vi "get image.vi"(8 "error in (no error)":errorcluster, 10 "previous buffer number":u32, 11 "image source data":T4) -> (0 "error out":errorcluster, 1 "aquisition time ms":u32, 2 "buffer number":u32, 3 "captured image":T1)   [LabVIEW 2013]
uses:
  <vilib>/userdefined/High Color/IMAQdx.ctl
  <vilib>/vision/Avi1.llb/AviRefnum.ctl
  <vilib>/vision/Image Controls.llb/IMAQ Image.ctl
  <vilib>/vision/driver/NI_Vision_Acquisition_Software.lvlib
  Image-Stack-Compressor/Stack Reader Wrapper/labview vis/StackReaderWrapper.lvlib
  <vilib>/vision/NI_Vision_Development_Module.lvlib
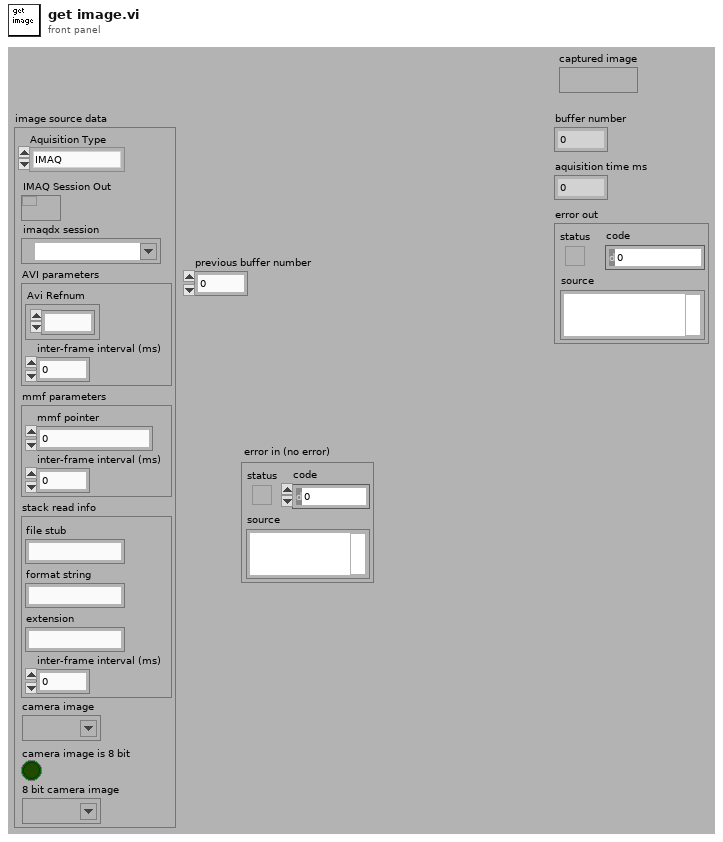
[diagram p1: front panel]
types:
  T1 = typedef "IMAQ Image.ctl" = refnum<image>
  T2 = typedef "IMAQdx.ctl" = refnum<k21>
  T3 = typedef "AviRefnum.ctl" = refnum<k1>
  T4 = cluster{"Aquisition Type":enum16{"IMAQ", "IMAQdx", "AVI", "MMF", "STACK"}, "IMAQ Session Out":refnum<k11>, "imaqdx session":T2, "AVI parameters":cluster{"Avi Refnum ":T3, "inter-frame interval (ms)":dbl}, "mmf parameters":cluster{"mmf pointer":u32, "inter-frame interval (ms)":dbl}, "stack read info":cluster{"file stub":string, "format string":string, "extension":string, "inter-frame interval (ms)":dbl}, "camera image":T1, "camera image is 8 bit":bool, "8 bit camera image":T1}
  T5 = cluster{"file stub":string, "format string":string, "extension":string, "inter-frame interval (ms)":dbl}
  T6 = typedef "Image Type" = u32
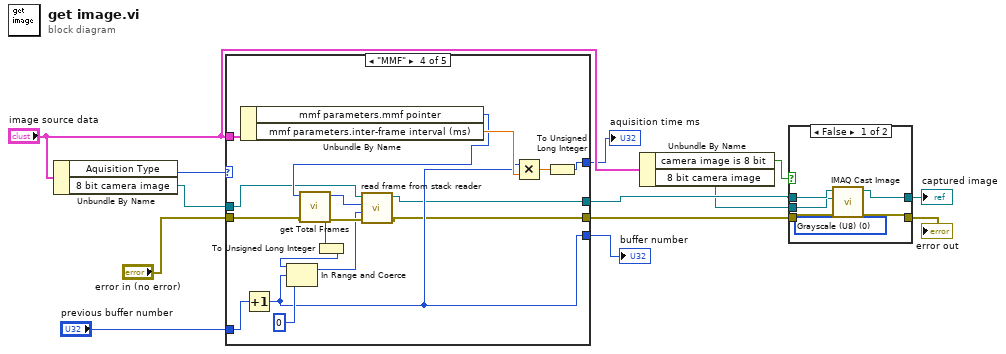
[diagram p0: block diagram]
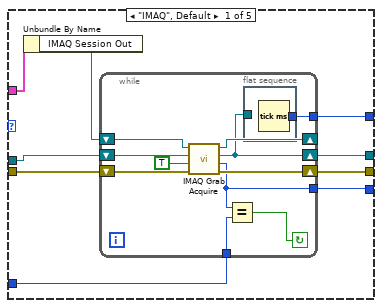
[diagram p3: hidden frame]
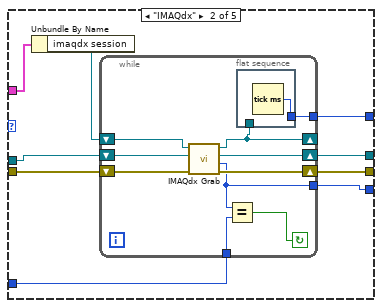
[diagram p4: hidden frame]
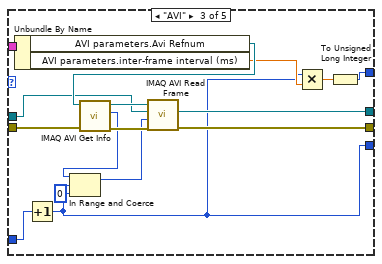
[diagram p5: hidden frame]
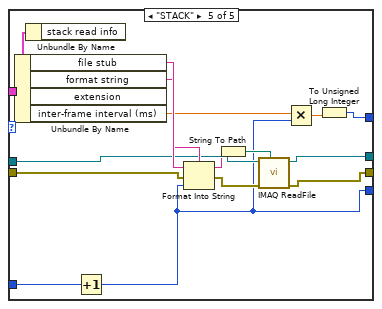
[diagram p6: hidden frame]
diagram:
  n1 = Unbundle By Name("image source data") -> ("Aquisition Type"=w13:enum16{"IMAQ", "IMAQdx", "AVI", "MMF", "STACK"}, "8 bit camera image"=w10:T1)
  n2 = case shown="\"MMF\"" w13 {
    tunnel: "image source data" -> [w17 w38 w70 w87 w103]
    tunnel: "error in (no error)" -> [w22 w43 w67 w80 w99]
    tunnel: [w21 w42 w59 w72 w93] -> w4
    tunnel: "previous buffer number" -> [w20 w41 w64 w86 w98]
    tunnel: [w19 w40 w60 w73 w92] -> w5
    tunnel: [w18 w39 w55 w81 w88] -> w7
    tunnel: w10 -> [w15 w36 w65 w76 w96]
    tunnel: [w14 w35 w57 w83 w90] -> w9
    frame "IMAQ", Default {
      n3 = Unbundle By Name(w17) -> ("IMAQ Session Out"=w16:refnum<k11>)
      n4 = while {
        shift-right: [w30] -> w21
        shift-left: w22 -> [w31]
        tunnel: w20 -> [w29]
        shift-right: [w25] -> w19
        shift-left: w15 -> [w32]
        tunnel: [w27] -> w18
        shift-right: [w26] -> _
        shift-left: w16 -> [w33]
        tunnel: [w24] -> w14
        stop <- w28 continue-if-true
        n5 = call <vilib>:"IMAQ Grab Acquire.vi"("error in (no error)"=w31, "Immediate?"=TRUE, "Image In"=w32, "IMAQ Session In"=w33) -> ("error out"=w30:errorcluster, "Acquired Buffer Number"=w24:u32, "Image Out"=w25:T1, "IMAQ Session Out"=w26:refnum<k11>)  [unwired: 4 in]
        n6 = Equal?(x=w24, y=w29) -> (x = y?=w28:bool)
        n7 = flat-sequence {
          tunnel: [w34] -> w27
          tunnel: w25 -> [_]
          frame #0 {
            n8 = Tick Count (ms)() -> (millisecond timer value=w34:u32)
          }
        }
      }
    }
    frame "IMAQdx" {
      n9 = Unbundle By Name(w38) -> ("imaqdx session"=w37:T2)
      n10 = while {
        shift-right: [w50] -> w42
        shift-left: w43 -> [w51]
        tunnel: w41 -> [w49]
        shift-right: [w47] -> w40
        shift-left: w36 -> [w52]
        tunnel: [w46] -> w39
        shift-right: [w45] -> _
        shift-left: w37 -> [w53]
        tunnel: [w44] -> w35
        stop <- w48 continue-if-true
        n11 = call <vilib>:"IMAQdx Grab.vi"("error in"=w51, "Image In"=w52, "Session In"=w53) -> ("error out"=w50:errorcluster, "Buffer Number Out"=w44:u32, "Image Out"=w47:T1, "Session Out"=w45:T2)  [unwired: 5 in]
        n12 = Equal?(x=w44, y=w49) -> (x = y?=w48:bool)
        n13 = flat-sequence {
          tunnel: [w54] -> w46
          tunnel: w45 -> [_]
          frame #0 {
            n14 = Tick Count (ms)() -> (millisecond timer value=w54:u32)
          }
        }
      }
    }
    frame "AVI" {
      n15 = Unbundle By Name(w70) -> ("AVI parameters.Avi Refnum"=w69:T3, "AVI parameters.inter-frame interval (ms)"=w58:dbl)
      n16 = Increment(x=w64) -> (x+1=w57:u32)
      n17 = call "IMAQ AVI Get Info"("error in (no error)"=w67, "Avi Refnum"=w69) -> ("error out"=w66:errorcluster, "Number of Frames"=w62:u32, "Avi Refnum (duplicate)"=w68:T3)  [unwired: 5 in, 2 out]
      n18 = In Range and Coerce(upper limit=w62, x=w57, lower limit=u32 0) -> (coerced(x)=w61:u32)  [unwired: 1 out]
      n19 = call "IMAQ AVI Read Frame"("error in (no error)"=w66, "Frame Number"=w61, "Image"=w65, "Avi Refnum"=w68) -> ("error out"=w59:errorcluster, "Image Out"=w60:T1)  [unwired: 4 in, 2 out]
      n20 = Multiply(x=w57, y=w58) -> (x*y=w56:dbl)
      n21 = To Unsigned Long Integer(number=w56) -> (unsigned 32bit integer=w55:u32)
    }
    frame "MMF" {
      n22 = Unbundle By Name(w87) -> ("mmf parameters.mmf pointer"=w79:u32, "mmf parameters.inter-frame interval (ms)"=w84:dbl)
      n23 = Increment(x=w86) -> (x+1=w83:u32)
      n24 = call "get Total Frames.vi"("error in (no error)"=w80, "sr"=w79) -> ("error out"=w77:errorcluster, "function return"=w78:i32, "sr out"=w75:u32)  [unwired: 7 in]
      n25 = To Unsigned Long Integer(number=w78) -> (unsigned 32bit integer=w71:u32)
      n26 = In Range and Coerce(upper limit=w71, x=w83, lower limit=u32 0) -> (coerced(x)=w74:u32)  [unwired: 1 out]
      n27 = call "read frame from stack reader.vi"("error in (no error)"=w77, "frameNumber"=w74, "sr"=w75, "image dst"=w76) -> ("error out"=w72:errorcluster, "Image Out"=w73:T1)  [unwired: 6 in]
      n28 = Multiply(x=w83, y=w84) -> (x*y=w82:dbl)
      n29 = To Unsigned Long Integer(number=w82) -> (unsigned 32bit integer=w81:u32)
    }
    frame "STACK" {
      n30 = Unbundle By Name(w103) -> ("stack read info"=w102:T5)
      n31 = Unbundle By Name(w102) -> ("file stub"=w101:string, "format string"=w100:string, "inter-frame interval (ms)"=w91:dbl)  [unwired: 1 out]
      n32 = Increment(x=w98) -> (x+1=w90:u32)
      n33 = Format Into String(format string=w100, initial string=w101, error in=w99, w90) -> (resulting string=w95:string, error out=w97:errorcluster)
      n34 = String To Path(string=w95) -> (path=w94:path)
      n35 = call "IMAQ ReadFile"("File Path"=w94, "error in (no error)"=w97, "Image"=w96) -> ("error out"=w93:errorcluster, "Image Out"=w92:T1)  [unwired: 4 in, 3 out]
      n36 = Multiply(x=w91, y=w90) -> (x*y=w89:dbl)
      n37 = To Unsigned Long Integer(number=w89) -> (unsigned 32bit integer=w88:u32)
    }
  }
  "buffer number" <- w9
  "aquisition time ms" <- w7
  n38 = Unbundle By Name("image source data") -> ("camera image is 8 bit"=w6:bool, "8 bit camera image"=w3:T1)
  n39 = case shown="False" w6 {
    tunnel: w5 -> [w107 w110]
    tunnel: w4 -> [w109 w111]
    tunnel: [w104 w111] -> w1
    tunnel: [w105 w110] -> w2
    tunnel: w3 -> [w106 _]
    frame False {
      w108 = T6 0 items=["Grayscale (U8)", "Grayscale (I16)", "Grayscale (SGL)", "Complex (CSG)", "RGB (U32)", "HSL (U32)", "RGB (U64)", "Grayscale (U16)"] ("Image Type")
      n40 = call "IMAQ Cast Image"("Image Type"=w108, "error in (no error)"=w109, "Image Dst"=w106, "Image Src"=w107) -> ("error out"=w104:errorcluster, "Image Dst Out"=w105:T1)  [unwired: 6 in]
    }
    frame True {
    }
  }
  "captured image" <- w2
  "error out" <- w1
